vi "meilhaus_voltage.vi"() -> ()   [LabVIEW 2009]
uses:
  <vilib>/ULx/Read.llb/ULx Read (Analog DBL 1Chan 1Samp).vi
  <vilib>/ULx/Create Channel.llb/ULx Create Channel (AO-Voltage-Basic).vi
  C:/Program Files (x86)/National Instruments/LabVIEW 2009/vi.lib/ULx/ULx_LV.dll
panel:
  out "NumberOfChannels":u32
  out "data":dbl format="%_6g"
  in  "physical channels":refnum<k21>
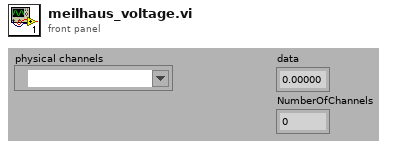
[diagram p1: front panel]
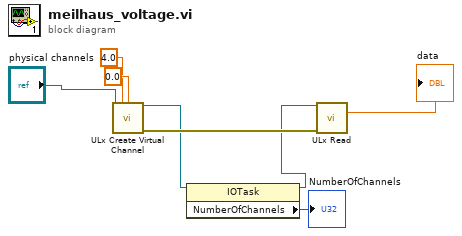
[diagram p0: block diagram]
diagram:
  n1 = call-poly <vilib>:"ULx Create Virtual Channel.vi"("maximum value"=4.0, "minimum value"=0.0, "physical channels"="physical channels") -> ("task out"=w2:refnum<k24>, "error out"=w4:errorcluster)  [unwired: 11 in]
  n2 = property class="IOTask"(reference=w2) -> (reference out=w1:refnum<k24>, "NumberOfChannels"=→"NumberOfChannels":u32)  [unwired: 1 in, 1 out]
  n3 = call-poly <vilib>:"ULx Read.vi"("task in"=w1, "error in"=w4) -> ("data"=→"data":dbl)  [unwired: 11 in, 2 out]
